vi "Get Target.vi"(8 "error in (no error)":errorcluster, 11 "Instrument.1820 in":refnum<class "Instrument.Oxford1820.lvclass">) -> (0 "error out":errorcluster, 1 "Target Field Rate (T/min)":dbl, 2 "Target Field (T)":dbl, 3 "Instrument.1820 in":refnum<class "Instrument.Oxford1820.lvclass">)   [LabVIEW 2019, in "Instrument.Oxford1820.lvclass"]
uses:
  Instrument.Oxford1820.lvclass
  Typedefs/PrivateEvents--Instrument.Oxford1820.setMagnet.ctl
  <userlib>/LevyLab/Instrument Framework/Instrument Types/Cryostat/Typedefs/Magnet Axis--Enum.ctl
  <userlib>/LevyLab/Instrument Framework/Instrument Types/Cryostat/Typedefs/Magnet Mode--Enum.ctl
  Typedefs/Instrument.Oxford1820.protectedCommands-enum.ctl
  2a741720-dfc8-4982-b19f-246f04608042.vi/5f521831-da7b-4adf-8ffa-6a8e3ceb4771.vi
  2a741720-dfc8-4982-b19f-246f04608042.vi/5f521831-da7b-4adf-8ffa-6a8e3ceb4771.vi/c0f20c47-3cd2-48cc-ad6b-3073082ccede.vi
  2a741720-dfc8-4982-b19f-246f04608042.vi/5f521831-da7b-4adf-8ffa-6a8e3ceb4771.vi/63d5b44f-7ae9-4b89-b19e-55a5311c25eb.vi
  <vilib>/Utility/Data Type/Get Type Information.vi
  <vilib>/JDP Science/JSONtext/JSON text to Variant.vi
  <vilib>/JDP Science/JSONtext/LVClass Serializer/JSONtext LVClass Serializer.lvclass
  <userlib>/LevyLab/Instrument Framework/Instrument Types/Cryostat/Instrument.Cryostat.lvclass
  89096aa0-db56-426b-8f4d-a59d04da8d42.vi
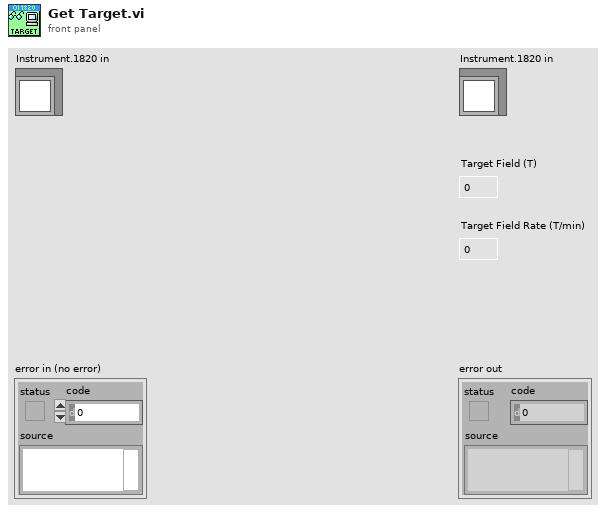
[diagram p1: front panel]
types:
  T1 = typedef "Instrument.Oxford1820.lvclass/Instrument.Oxford1820.protectedCommands-enum.ctl" = enum16{"Hold", "RampToSet", "RampToZero", "Clamp", "setTarget", "setSwitchHeat", "setLambda", "setFillMode", "setNeedleValve", "getStatus", "getTarget", "getSwitchHeat", "getPSUField", "setSequenceStatus"}
  T2 = typedef "Instrument.Oxford1820.lvclass/PrivateEvents--Instrument.Oxford1820.setMagnet.ctl" = cluster{"field":dbl, "rate":dbl, "axis":T3, "mode":T4}
  T3 = typedef "Instrument.Cryostat.lvclass/Magnet Axis--Enum.ctl" = enum16{"X", "Y", "Z"}
  T4 = typedef "Instrument.Cryostat.lvclass/Magnet Mode--Enum.ctl" = enum16{"Persistent", "Driven"}
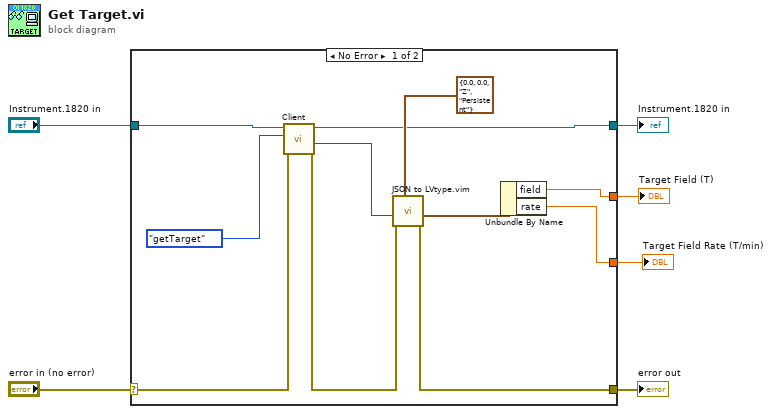
[diagram p0: block diagram]
diagram:
  n1 = case shown="No Error" "error in (no error)" {
    selector: "error in (no error)" -> [w12 w19]
    tunnel: [w11 w19] -> w5
    tunnel: [w7 w18] -> w3
    tunnel: "Instrument.1820 in" -> [w13 w18]
    tunnel: [w17 _] -> w2
    tunnel: [w16 _] -> w1
    frame No Error {
      n2 = call-dynamic "Client.vi"("error in (no error)"=w12, "Command in"=Instrument.Oxford1820.protectedCommands-enum."getTarget" ("Commands"), "Instrument in"=w13) -> ("error out"=w10:errorcluster, "Data out"=w15:variant, "Instrument out"=w7:refnum<class "Instrument.Oxford1820.lvclass">)  [unwired: 5 in, 1 out]
      n3 = call "JSON to LVtype.vim"("type"=T2 {"field"=0.0, "rate"=0.0, "axis"=enum."Z", "mode"=enum."Persistent"} ("Set Magnet Field"), "error in (no error)"=w10, "JSON Data in"=w15) -> ("error out"=w11:errorcluster, "Data out"=w9:T2)  [unwired: 7 in]
      n4 = Unbundle By Name(w9) -> ("field"=w17:dbl, "rate"=w16:dbl)
    }
    frame Error {
    }
  }
  "error out" <- w5
  "Instrument.1820 in" <- w3
  "Target Field (T)" <- w2
  "Target Field Rate (T/min)" <- w1
